vi "test_VISA Write.vi"(8 "error in (no error)":errorcluster, 11 "TestCase in":refnum<class "Instrument Addon Serial Protocols Unit Tests.lvclass">) -> (0 "error out":errorcluster, 3 "TestCase out":refnum<class "Instrument Addon Serial Protocols Unit Tests.lvclass">)   [LabVIEW 2023, in "Instrument Addon Serial Protocols Unit Tests.lvclass"]
uses:
  Instrument Addon Serial Protocols Unit Tests.lvclass
  Instrument Addon Serial Protocols Unit Tests.lvclass/Instrument Addon Serial Protocols Unit Tests.ctl
  <vilib>/addons/_JKI Toolkits/VI Tester/TestCase.llb/TestCase.lvclass
  VISA/VISA.lvclass
  Listener/Listener.lvclass
  Listener/ListenerClassControls/Operation.ctl
  <vilib>/platform/TimedLoop/XDataNode/XDataNode.xnode
  <vilib>/Platform/TimedLoop/XDataNode/nitl_modes.ctl
  <vilib>/Platform/TimedLoop/XDataNode/XDNodeRunTimeDep.lvlib
  <vilib>/Platform/TimedLoop/XDataNode/wakeup.ctl
  <vilib>/Platform/TimedLoop/XDataNode/timing_clust.ctl
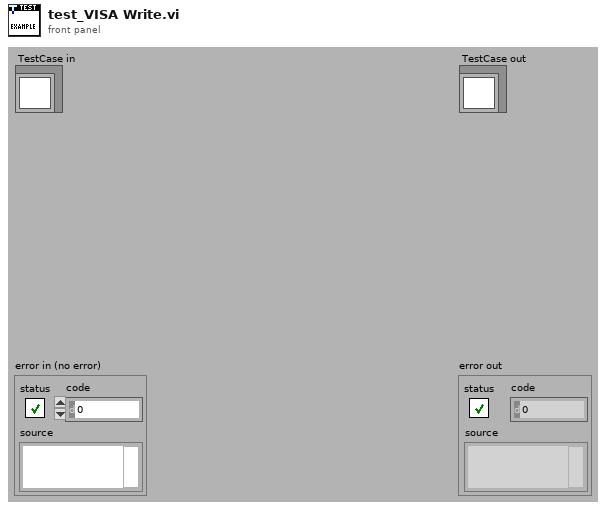
[diagram p1: front panel]
types:
  T1 = typedef "Listener.lvclass/Operation.ctl" = enum16{"Read", "Write"}
  T2 = typedef "XDNodeRunTimeDep.lvlib/timing_clust.ctl" = cluster{"Expected End [f-1]":u64, "Actual End [f-1]":u64, "Finished Late? [f-1]":bool, "Expected End [i-1]":u64, "Actual End [i-1]":u64, "Finished Late? [i-1]":bool, "Expected Start [i]":u64, "Actual Start [i]":u64, "Expected Start [f]":u64, "Actual Start [f]":u64, "Source Name":string, "Structure Name":string, "Period":i64, "Deadline":i64, "Offset":i64, "Start":i64, "Priority":i32, "Timeout":i32, "Mode":T3, "Wakeup Reason":T4, "Error":errorcluster, "Source Type":string, "Secondary Source Type":string, "Global End Time":u64, "Global Start Time":u64, "Frame Duration":u64, "Iteration Duration":u64, "Assigned CPU":i32, "I/O Scan Engine Mode":u32}
  T3 = typedef "XDNodeRunTimeDep.lvlib/nitl_modes.ctl" = enum32{"No Change", "Process missed periods, maintain original phase", "Discard missed periods, maintain original phase", "Process missed periods, ignore original phase", "Discard missed periods, ignore original phase"}
  T4 = typedef "XDNodeRunTimeDep.lvlib/wakeup.ctl" = enum32{"Normal", "Aborted", "Asynchronous wakeup", "Timing source error", "Timed loop error", "Timeout"}
  T5 = typedef "Listener.lvclass/VISA Data Structure.ctl" = cluster{"Data Length":u32, "Data":string}
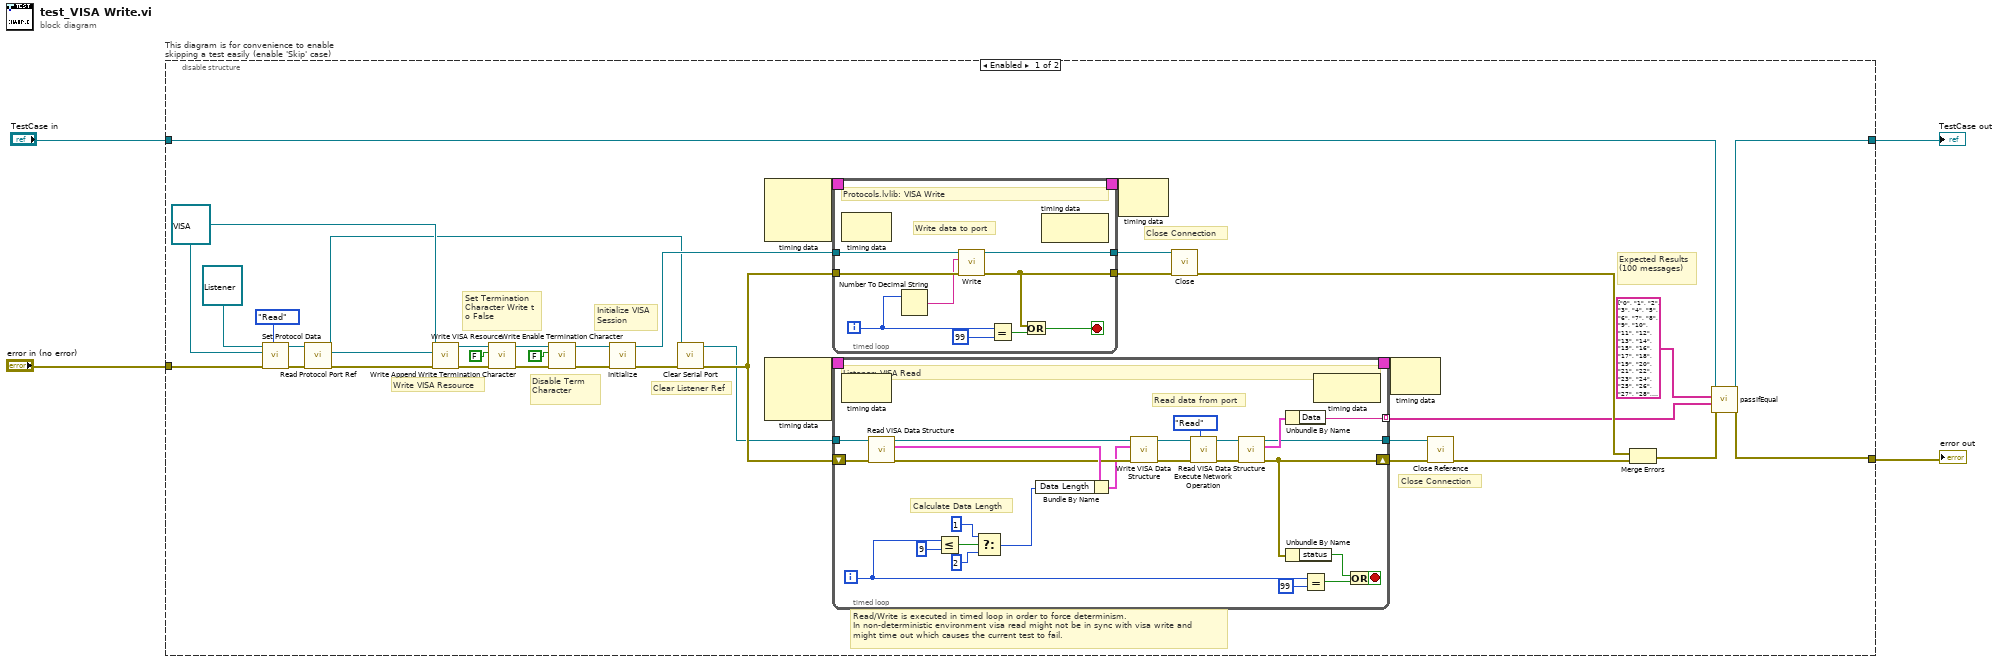
[diagram p0: block diagram]
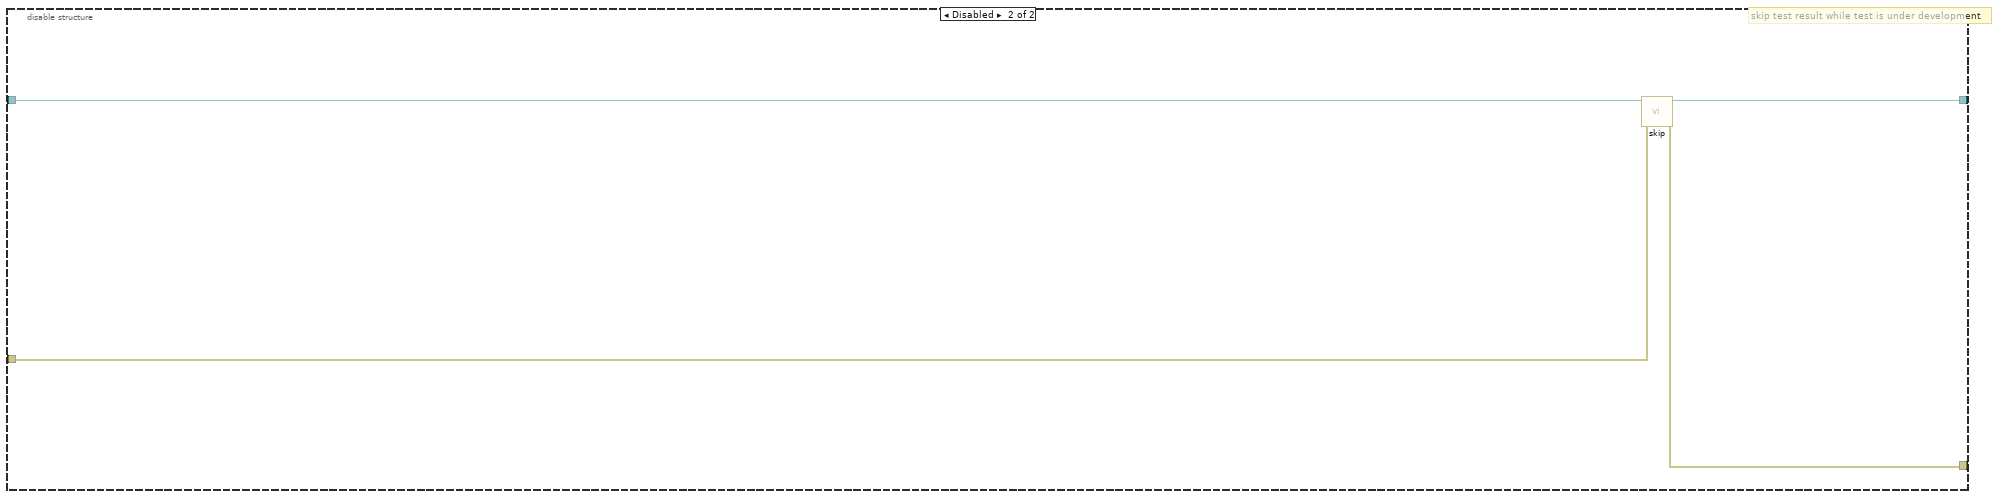
[diagram p2: hidden frame]
diagram:
  n1 = disable-structure "This diagram is for convenience to enable skipping a test easily (enable 'Skip' case)" shown="Enabled" {
    disable-tunnel: "TestCase in" -> [w41 w87]
    disable-tunnel: [w40 w85] -> w1
    disable-tunnel: [w39 w86] -> w3
    disable-tunnel: "error in (no error)" -> [w35 w84]
    frame Enabled {
      w25 = refnum<class "VISA.lvclass"> refnum ("Protocols.lvlib:VISA.lvclass")
      # "Clear Listener Ref"
      # "Initialize VISA\nSession"
      # "Disable Term\nCharacter"
      # "Set Termination \nCharacter Write t\no False"
      # "Write VISA Resource"
      # "Close Connection"
      # "Close Connection"
      # "Read/Write is executed in timed loop in order to force determinism.\nIn non-deterministic environment visa read might not be in sync with visa write and\nmight time out which causes the current test to fail."
      # "Expected Results\n(100 messages)"
      n2 = call "Set Protocol Data.vi"("Operation"=Operation."Read", "error in (no error)"=w35, "Protocols.lvlib:Protocol Parent.lvclass"=w25, "Listener In.lvclass"=refnum<class "Listener.lvclass"> refnum ("Listener.lvclass")) -> ("error out"=w9:errorcluster, "Listener Out.lvclass"=w8:refnum<class "Listener.lvclass">)  [unwired: 6 in]
      n3 = call "Read Protocol Port Ref.vi"("error in (no error)"=w9, "Listener in"=w8) -> ("error out"=w7:errorcluster, "Protocol Port Ref"=w6:refnum<visa-resource-name>, "Listener out"=w5:refnum<class "Listener.lvclass">)  [unwired: 7 in]
      n4 = call "Write VISA Resource.vi"("error in (no error)"=w7, "VISA Resource"=w6, "VISA in"=w25) -> ("error out"=w26:errorcluster, "VISA out"=w27:refnum<class "VISA.lvclass">)  [unwired: 7 in]
      n5 = call "Write Append Write Termination Character.vi"("error in (no error)"=w26, "Append Write Termination Character"=FALSE, "VISA in"=w27) -> ("error out"=w30:errorcluster, "VISA out"=w29:refnum<class "VISA.lvclass">)  [unwired: 7 in]
      n6 = call "Write Enable Termination Character.vi"("error in (no error)"=w30, "Enable Termination Character"=FALSE, "VISA in"=w29) -> ("error out"=w18:errorcluster, "VISA out"=w20:refnum<class "VISA.lvclass">)  [unwired: 7 in]
      n7 = call-dynamic "Initialize.vi"("error in (no error)"=w18, "VISA in"=w20) -> ("error out"=w13:errorcluster, "VISA out"=w19:refnum<class "VISA.lvclass">)  [unwired: 8 in]
      n8 = call "Clear Serial Port.vi"("error in (no error)"=w13, "Listener In.lvclass"=w5) -> ("error out"=w12:errorcluster, "Listener out"=w11:refnum<class "Listener.lvclass">)  [unwired: 8 in]
      n9 = node-c288() -> (w17:T2)  [unwired: 3 in]
      n10 = node-c288() -> (w15:T2)  [unwired: 3 in]
      n11 = timed-loop {
        tunnel: w19 -> [w78]
        tunnel: [w77] -> w23
        timing: w17 -> [_]
        timing-out: [_] -> w16
        tunnel: w12 -> [w79]
        tunnel: [w74] -> w24
        i -> [w73]
        stop <- w71 stop-if-true
        # "Write data to port"
        # "Protocols.lvlib: VISA Write"
        n12 = node-c288() -> ()  [unwired: 1 in, 1 out]
        n13 = Number To Decimal String(number=w73) -> (decimal integer string=w76:string)  [unwired: 1 in]
        n14 = call-dynamic "Write.vi"("error in (no error)"=w79, "String"=w76, "VISA in"=w78) -> ("error out"=w74:errorcluster, "VISA out"=w77:refnum<class "VISA.lvclass">)  [unwired: 7 in]
        n15 = Equal?(x=w73, y=99) -> (x = y?=w75:bool)
        n16 = Or(x=w74, y=w75) -> (x .or. y?=w71:bool)
        n17 = node-c288() -> ()  [unwired: 1 in, 1 out]
      }
      n18 = timed-loop {
        shift-right: [w43] -> w21
        shift-left: w12 -> [w52]
        tunnel: w11 -> [w51]
        tunnel: [w63] -> w22
        tunnel: [w62] -> w32 mode=indexing
        timing: w15 -> [_]
        timing-out: [_] -> w14
        i -> [w44]
        stop <- w58 stop-if-true
        # "Calculate Data Length"
        # "Read data from port"
        # "Listener: VISA Read"
        n19 = node-c288() -> ()  [unwired: 1 in, 1 out]
        n20 = call-dynamic "Read VISA Data Structure.vi"("error in (no error)"=w52, "Listener in"=w51) -> ("error out"=w48:errorcluster, "VISA Data Structure"=w50:T5, "Listener out"=w47:refnum<class "Listener.lvclass">)  [unwired: 7 in]
        n21 = Less Or Equal?(x=w44, y=9) -> (x <= y?=w56:bool)
        n22 = Select(t=u32 1 ("y"), s=w56, f=u32 2) -> (s? t:f=w53:u32)
        n23 = Bundle By Name(cluster=w50, "Data Length"=w53) -> (w45:T5)
        n24 = call-dynamic "Write VISA Data Structure.vi"("error in (no error)"=w48, "VISA Data Structure"=w45, "Listener in"=w47) -> ("error out"=w49:errorcluster, "Listener out"=w46:refnum<class "Listener.lvclass">)  [unwired: 7 in]
        n25 = call "Execute Network Operation.vi"("Operation"=Operation."Read", "error in (no error)"=w49, "Listener In.lvclass"=w46) -> ("error out"=w65:errorcluster, "Listener Out.lvclass"=w66:refnum<class "Listener.lvclass">)  [unwired: 7 in]
        n26 = call-dynamic "Read VISA Data Structure.vi"("error in (no error)"=w65, "Listener in"=w66) -> ("error out"=w43:errorcluster, "VISA Data Structure"=w64:T5, "Listener out"=w63:refnum<class "Listener.lvclass">)  [unwired: 7 in]
        n27 = Unbundle By Name(w64) -> ("Data"=w62:string)
        n28 = Unbundle By Name(w43) -> ("status"=w42:bool)
        n29 = Equal?(x=w44, y=99) -> (x = y?=w59:bool)
        n30 = node-c288() -> ()  [unwired: 1 in, 1 out]
        n31 = Or(x=w42, y=w59) -> (x .or. y?=w58:bool)
      }
      n32 = node-c288(w16) -> ()  [unwired: 1 out]
      n33 = call-dynamic "Close.vi"("error in (no error)"=w24, "VISA in"=w23) -> ("error out"=w34:errorcluster)  [unwired: 8 in, 1 out]
      n34 = node-c288(w14) -> ()  [unwired: 1 out]
      n35 = call "Close Reference.vi"("error in (no error)"=w21, "Listener In.lvclass"=w22) -> ("error out"=w33:errorcluster)  [unwired: 8 in, 1 out]
      n36 = Merge Errors(w34, w33) -> (w36:errorcluster)
      n37 = call-dynamic "passIfEqual.vi"("error in (no error)"=w36, "y"=w32, "x"=string[] ["0", "1", "2", "3", "4", "5", "6", "7", "8", "9", "10", "11", "12", "13", "14", "15", "16", "17", "18", "19", "20", "21", "22", "23", "24", "25", "26", "27", "28", "29", "30", "31", "32", "33", "34", "35", "36", "37", "38", "39", "40", "41", "42", "43", "44", "45", "46", "47", "48", "49", "50", "51", "52", "53", "54", "55", "56", "57", "58", "59", "60", "61", "62", "63", "64", "65", "66", "67", "68", "69", "70", "71", "72", "73", "74", "75", "76", "77", "78", "79", "80", "81", "82", "83", "84", "85", "86", "87", "88", "89", "90", "91", "92", "93", "94", "95", "96", "97", "98", "99"] ("Array"), "TestCase in"=w41) -> ("error out"=w39:errorcluster, "TestCase out"=w40:refnum<class "Instrument Addon Serial Protocols Unit Tests.lvclass">)  [unwired: 6 in]
    }
    frame Disabled {
      # "skip test result while test is under development"
      n38 = call <vilib>:"skip.vi"("error in (no error)"=w84, "TestCase in"=w87) -> ("error out"=w86:errorcluster, "TestCase out"=w85:refnum<class "Instrument Addon Serial Protocols Unit Tests.lvclass">)  [unwired: 8 in]
    }
  }
  "error out" <- w3
  "TestCase out" <- w1
